vi "Scan_Addresses_and_Return_DeviceInfo.vi"() -> ()   [LabVIEW 2017]
uses:
  U:/UDocuments/Thorlabs.Elliptec.ELLO_DLL.dll
  Thorlabs.Elliptec.ELLO_DLL.dll
panel:
  out "Device Information in Bytes":string[](array[string])
  out "Device Description":string[][](array[string])
  out "Number of Detected Devices":i32
  # "Notes:"
  # "This VI does not require you to use specific hardware. Any elliptec device is compatible and can they can be running \"Daisy-Chained\" \nor through the ELLB Control Bus Distributor. The maximum number of devices it can search through on a single COM port is 16.\nThe stages can not share the same address as this will cause confusion and only one device will be displayed, with a serial number \nwhich corresponds to neither stage.\n\nIf, when running the VI for the first time, you get a popup as illustrated below, then click Browse and navigate to the \nThorlabs.Elliptec.ELLO_DLL.dll file in the ELLO software installation directory. This can be copied to the folder you are \nrunning the VI from."
  # "Thorlabs Hardware: ELL6, ELL9, ELL14, ELL17, ELL18, ELLB \nhttps://www.thorlabs.com/thorproduct.cfm?partnumber=ELL17\n\nDescription: This VI will enable you to search for connected devices at the COM port of your choosing and extract the characterising information about that stage. It does not matter which ELL hardware has been connected."
  # "Instructions:"
  # "1) Connect your devices to the USB Interface board via the ribbon cable. \n2) Connect power to the board and wait for approximately 15 seconds. As soon as the stage has power it will attempt a frequency search.\n     If the power is insufficient the board will not find the correct operating frequencies. This is why the USB is attached last. Ensure   \n     sufficient current is supplied for the number of attached stages.\n3) Connect the interface board to the PC via the USB cable.\n4) Run the VI."
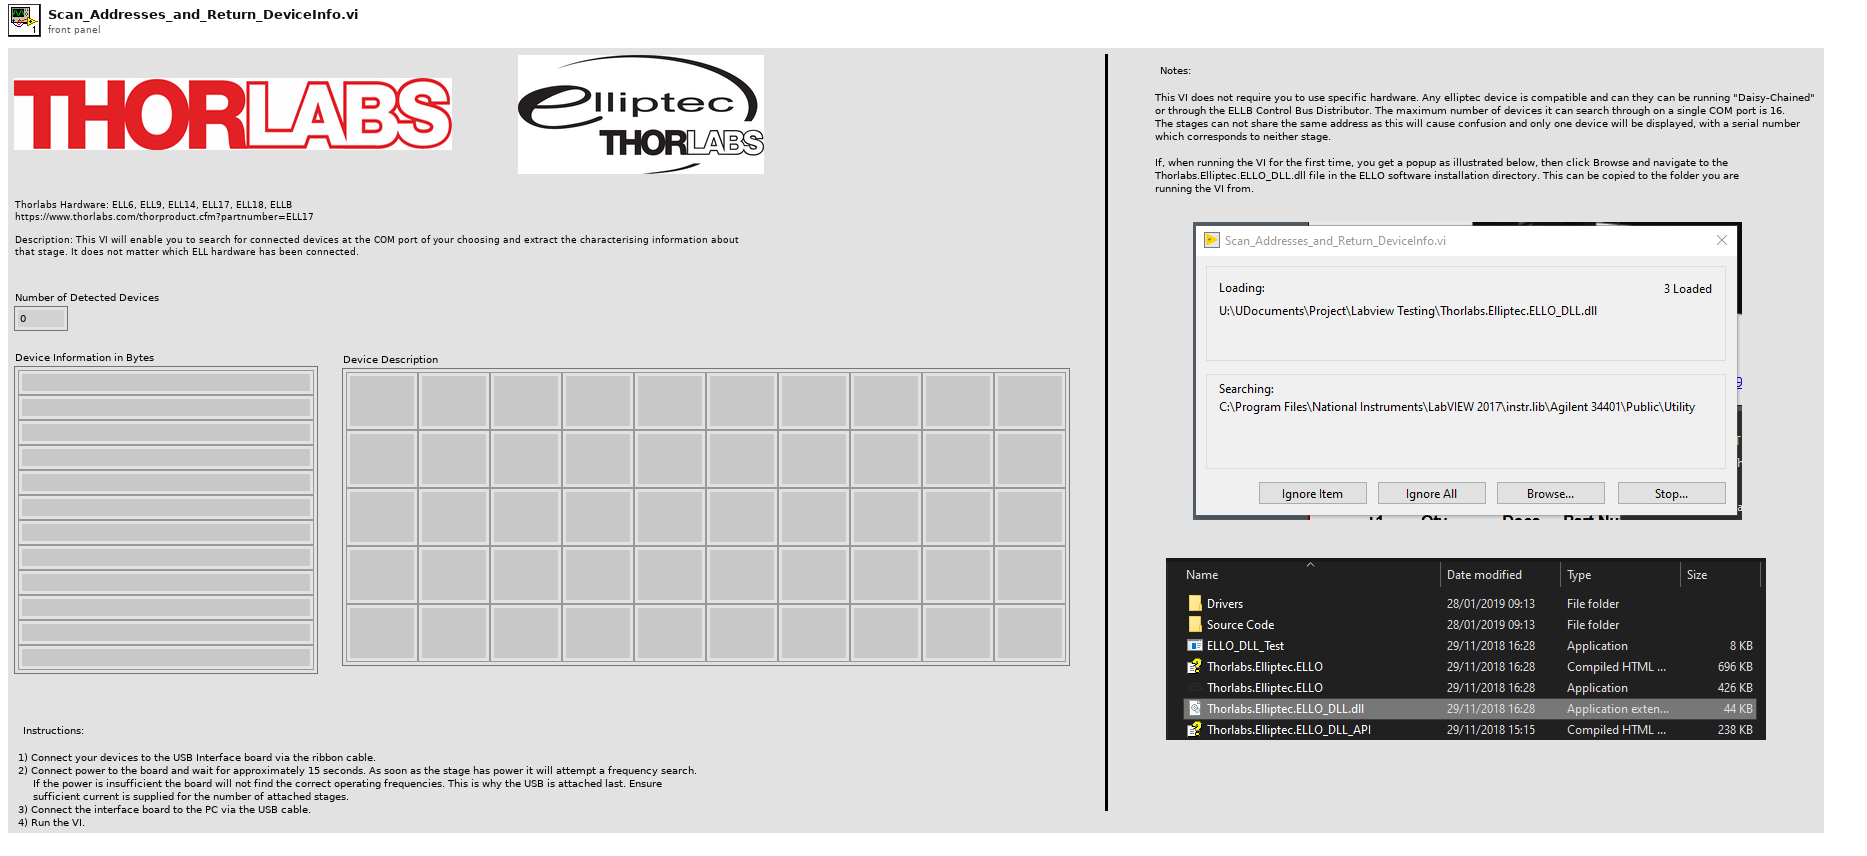
[diagram p1: front panel]
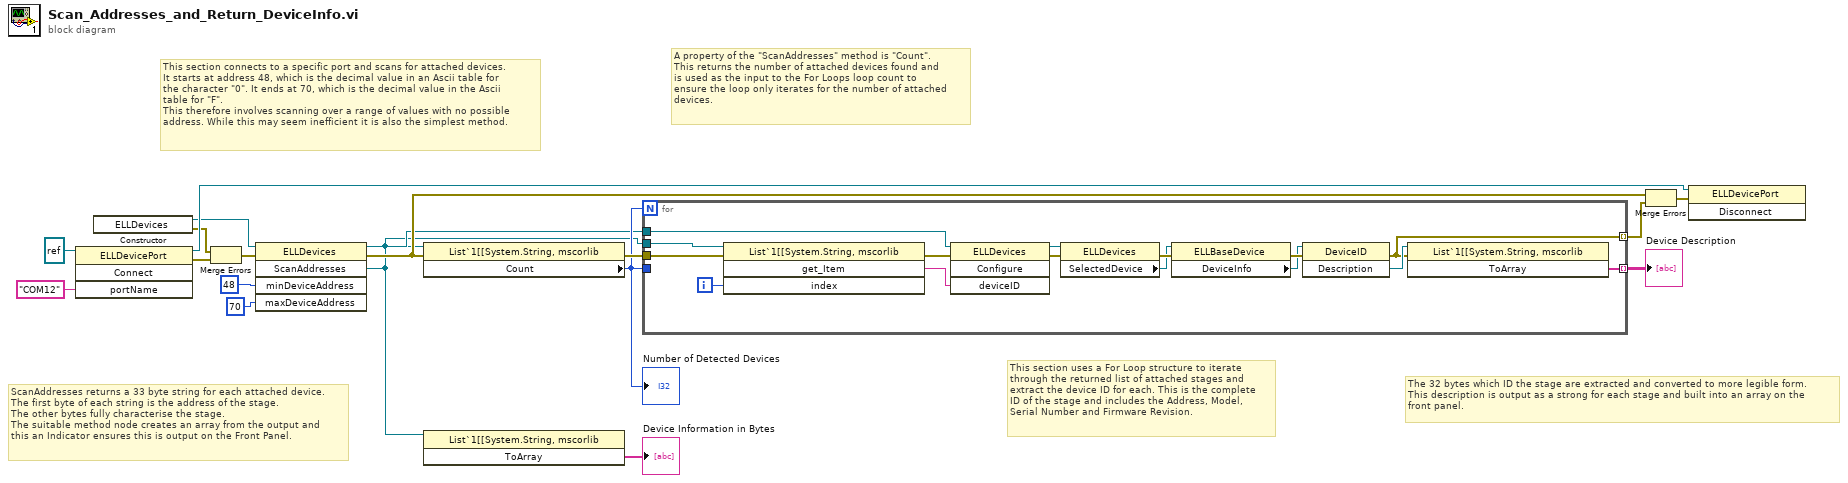
[diagram p0: block diagram]
diagram:
  # "The 32 bytes which ID the stage are extracted and converted to more legible form.\nThis description is output as a strong for each stage and built into an array on the\nfront panel."
  # "ScanAddresses returns a 33 byte string for each attached device.\nThe first byte of each string is the address of the stage.\nThe other bytes fully characterise the stage.\nThe suitable method node creates an array from the output and\nthis an Indicator ensures this is output on the Front Panel."
  # "A property of the \"ScanAddresses\" method is \"Count\". \nThis returns the number of attached devices found and\nis used as the input to the For Loops loop count to\nensure the loop only iterates for the number of attached\ndevices."
  # "This section connects to a specific port and scans for attached devices.\nIt starts at address 48, which is the decimal value in an Ascii table for\nthe character \"0\". It ends at 70, which is the decimal value in the Ascii\ntable for \"F\".\nThis therefore involves scanning over a range of values with no possible\naddress. While this may seem inefficient it is also the simplest method."
  # "This section uses a For Loop structure to iterate \nthrough the returned list of attached stages and \nextract the device ID for each. This is the complete\nID of the stage and includes the Address, Model,\nSerial Number and Firmware Revision."
  n1 = invoke class="ELLDevicePort" method="Connect"(reference=refnum<k24> refnum, "portName"="COM12") -> (reference out=w17:refnum<k24>, error out=w11:errorcluster)  [unwired: 2 in, 2 out]
  n2 = constructor class="ELLDevices"() -> (reference out=w15:refnum<k24>, error out=w12:errorcluster)  [unwired: 3 in, 1 out]
  n3 = Merge Errors(w12, w11) -> (w10:errorcluster)
  n4 = invoke class="ELLDevices" method="ScanAddresses"(reference=w15, error in=w10, "minDeviceAddress"=u16 48, "maxDeviceAddress"=u16 70) -> (reference out=w4:refnum<k24>, error out=w8:errorcluster, "ScanAddresses"=w2:refnum<k24>)  [unwired: 1 in, 2 out]
  n5 = property class="List`1[[System.String, mscorlib"(reference=w2, error in=w8) -> (error out=w9:errorcluster, "Count"=w5:i32)  [unwired: 1 out]
  "Number of Detected Devices" <- w5
  n6 = invoke class="List`1[[System.String, mscorlib" method="ToArray"(reference=w2) -> ("ToArray"=→"Device Information in Bytes":string[])  [unwired: 2 in, 2 out]
  n7 = for {
    N: w5 -> [_]
    tunnel: w9 -> [w25]
    tunnel: [w20] -> w7 mode=indexing
    tunnel: w2 -> [w24]
    tunnel: w5 -> [_]
    tunnel: w4 -> [w22]
    tunnel: [w19] -> w1 mode=indexing
    i -> [w26]
    n8 = invoke class="List`1[[System.String, mscorlib" method="get_Item"(reference=w24, error in=w25, "index"=w26) -> (error out=w30:errorcluster, "get_Item"=w23:string)  [unwired: 1 in, 2 out]
    n9 = invoke class="ELLDevices" method="Configure"(reference=w22, error in=w30, "deviceID"=w23) -> (reference out=w27:refnum<k24>, error out=w31:errorcluster)  [unwired: 1 in, 2 out]
    n10 = property class="ELLDevices"(reference=w27, error in=w31) -> (error out=w32:errorcluster, "SelectedDevice"=w28:refnum<k24>)  [unwired: 1 out]
    n11 = property class="ELLBaseDevice"(reference=w28, error in=w32) -> (error out=w33:errorcluster, "DeviceInfo"=w29:refnum<k24>)  [unwired: 1 out]
    n12 = invoke class="DeviceID" method="Description"(reference=w29, error in=w33) -> (error out=w20:errorcluster, "Description"=w21:refnum<k24>)  [unwired: 1 in, 1 out]
    n13 = invoke class="List`1[[System.String, mscorlib" method="ToArray"(reference=w21, error in=w20) -> ("ToArray"=w19:string[])  [unwired: 1 in, 2 out]
  }
  "Device Description" <- w1
  n14 = Merge Errors(w8, w7) -> (w6:errorcluster)
  n15 = invoke class="ELLDevicePort" method="Disconnect"(reference=w17, error in=w6) -> ()  [unwired: 1 in, 3 out]
